vi "FaulhaberobjectsTextlist.vi"() -> ()   [LabVIEW 2011]
uses:
  FaulaberType.ctl
  FaulhaberAccess.ctl
panel:
  out "String":string
  out "Faulhaber Objects":T3(array[cluster]) {"ID" format="%x"}
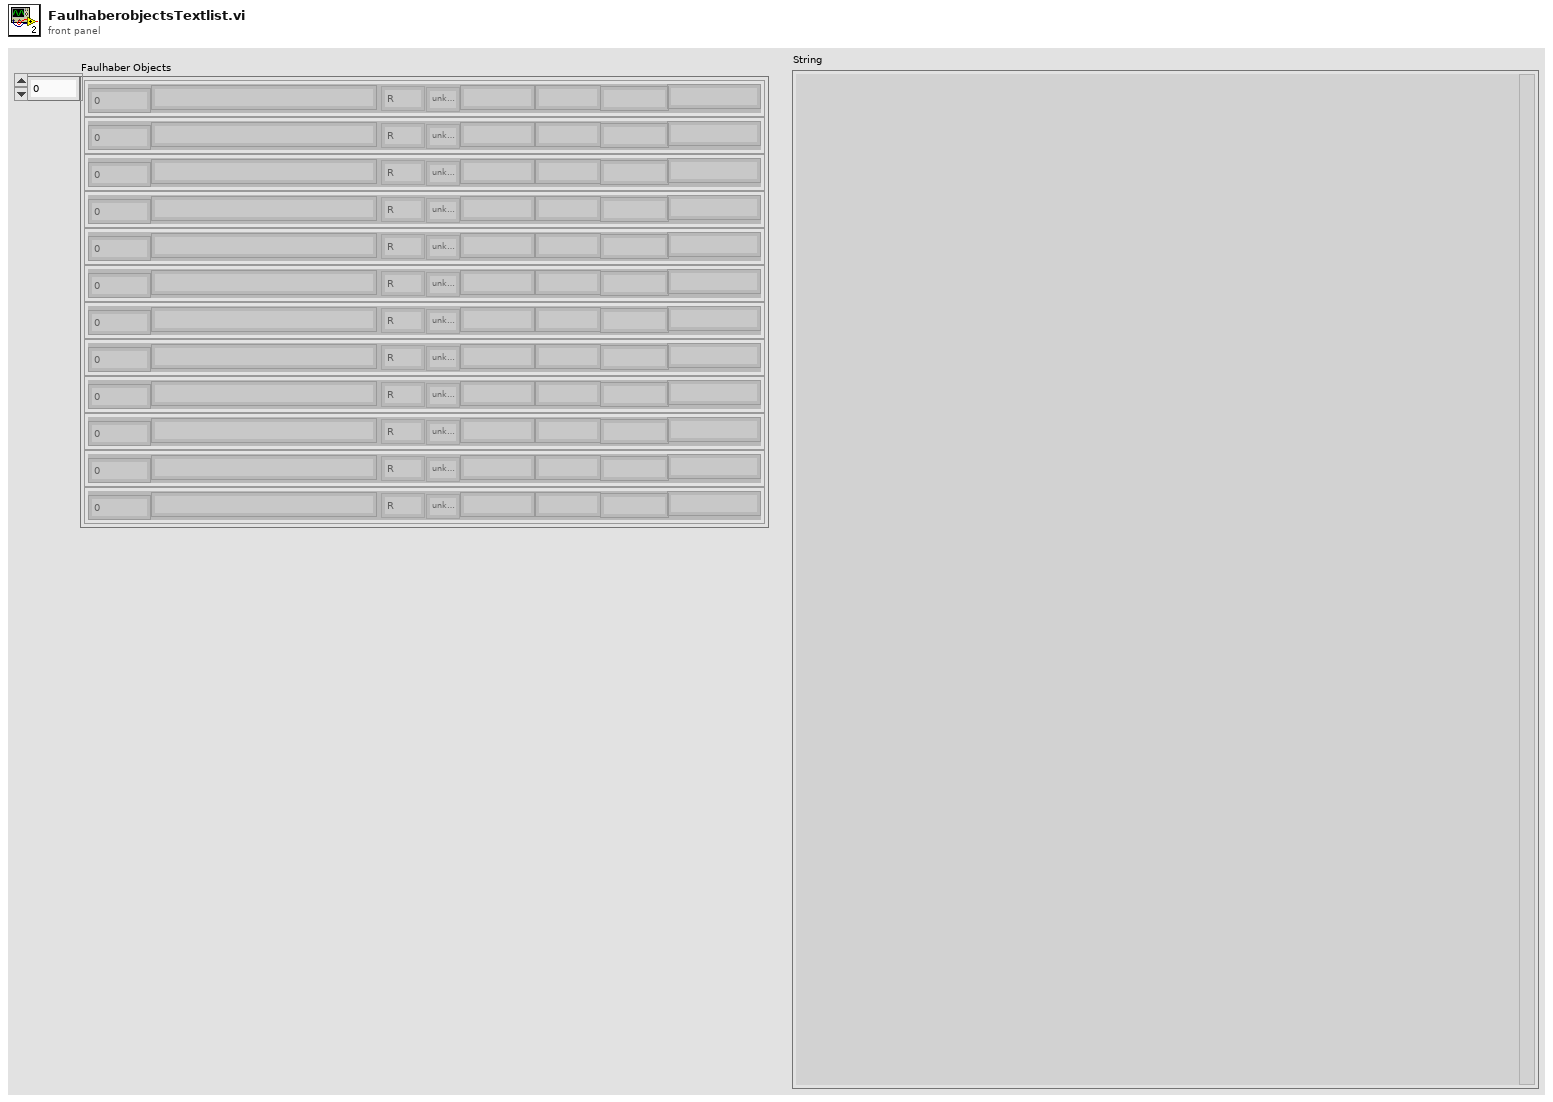
[diagram p1: front panel]
types:
  T1 = typedef "FaulaberType.ctl" = enum8{"unknown", "none", "S8", "S16", "S32", "U8", "U16", "U32", "R", "string"}
  T2 = typedef "FaulhaberAccess.ctl" = enum16{"unknown", "ro", "rw", "wo", "const"}
  T3 = cluster{"ID":u32, "Name":string, "type":T1, "rw":T2, "lowLimit":string, "highLimit":string, "Default":string, "Kommentart":string}[]
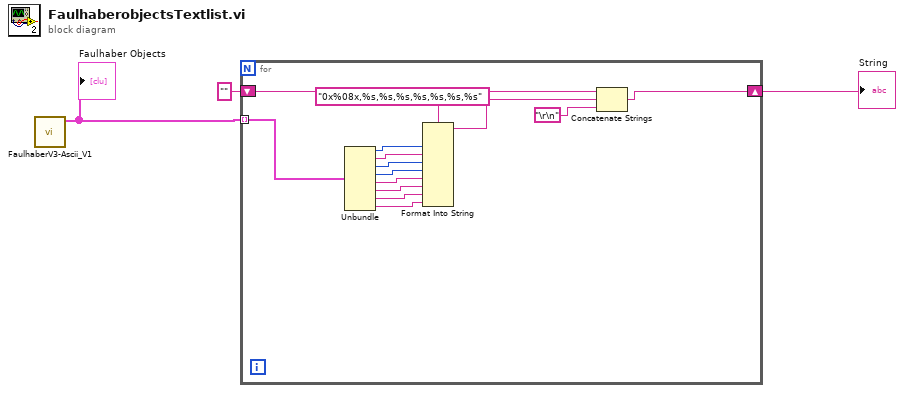
[diagram p0: block diagram]
diagram:
  n1 = call "FaulhaberV3-Ascii_V1.vi"() -> ("Faulhaber Objects"=w3:T3)  [unwired: 9 in, 2 out]
  "Faulhaber Objects" <- w3
  n2 = for {
    tunnel: w3 -> [w17] mode=indexing
    shift-right: [w15] -> w1
    shift-left: "" -> [w16]
    n3 = Unbundle(w17) -> ("ID"=w14:u32, "Name"=w13:string, "type"=w12:T1, "rw"=w11:T2, "lowLimit"=w10:string, "highLimit"=w9:string, "Default"=w8:string, "Kommentart"=w7:string)
    n4 = Format Into String(format string="0x%08x,%s,%s,%s,%s,%s,%s,%s", w14, w13, w12, w11, w10, w9, w8, w7) -> (resulting string=w5:string)  [unwired: 2 in, 1 out]
    n5 = Concatenate Strings(w16, w5, "\r\n") -> (w15:string)
  }
  "String" <- w1
